vi "New.vi"(6 "Delimiters":T1={"Close"="}}", "Open"="{{"}, 8 "Error In":errorcluster, 11 "Content":string) -> (0 "Error Out":errorcluster, 3 "Comment":refnum<class "Comment.lvclass">)   [LabVIEW 2018, in "Toolkit.lvlib" / "Nodes.lvlib" / "Comment.lvclass"]
doc: "Creates a new Comment node that represents a Mustache Comment tag in a parsed template."
uses:
  Comment.lvclass
  Type Definitions/Delimiters.ctl
  Comment.lvclass/Comment.ctl
  Toolkit.lvlib
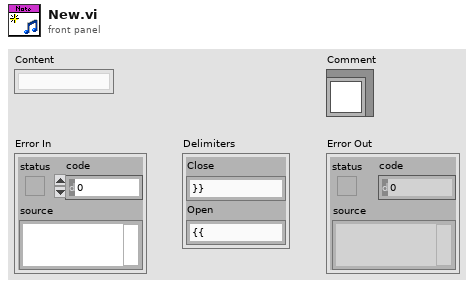
[diagram p1: front panel]
types:
  T1 = typedef "Toolkit.lvlib/Delimiters.ctl" = cluster{"Close":string, "Open":string}
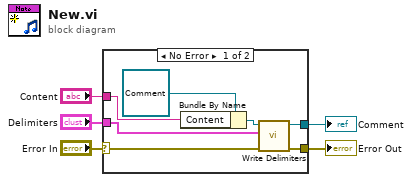
[diagram p0: block diagram]
diagram:
  n1 = case shown="No Error" "Error In" {
    selector: "Error In" -> [w12 w13]
    tunnel: [w10 w13] -> w4
    tunnel: "Content" -> [w11 _]
    tunnel: [w7 _] -> w2
    tunnel: "Delimiters" -> [w6 _]
    frame No Error {
      n2 = Bundle By Name(cluster=refnum<class "Comment.lvclass"> refnum ("Toolkit.lvlib:Nodes.lvlib:Comment.lvclass"), "Content"=w11) -> (w8:refnum<class "Comment.lvclass">)
      n3 = call-dynamic "Write Delimiters.vi"("Error In"=w12, "Delimiters"=w6, "Node In"=w8) -> ("Error Out"=w10:errorcluster, "Node Out"=w7:refnum<class "Comment.lvclass">)  [unwired: 7 in]
    }
    frame Error {
    }
  }
  "Comment" <- w2
  "Error Out" <- w4
